vi "Graph.vi"(4 "Resistance":dbl[](array[numeric]), 6 "Array in":T2(array[cluster]), 8 "error in (no error)":errorcluster, 9 "T  (ºC)":dbl format="%.2g", 10 "RH  (%)":dbl format="%.2g", 11 "Ethanol (%)":dbl format="%.3g") -> (0 "error out":errorcluster, 3 "Cluster":T1)   [LabVIEW 2020]
uses:
  typeDefs/Graph.ctl
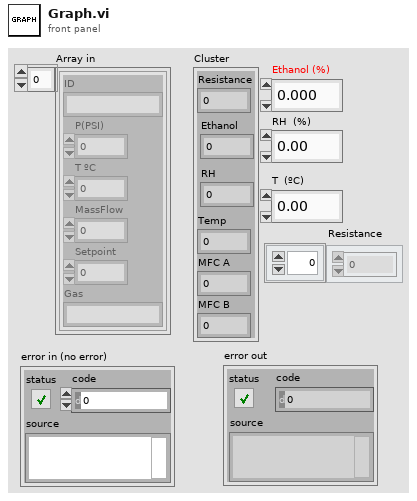
[diagram p1: front panel]
types:
  T1 = typedef "Graph.ctl" = cluster{"Resistance":dbl, "Ethanol":dbl, "RH":dbl, "Temp":dbl, "MFC A":dbl, "MFC B":dbl}
  T2 = cluster{"ID":string, "P(PSI)":dbl, "T ºC":dbl, "MassFlow":dbl, "Setpoint":dbl, "Gas":string}[]
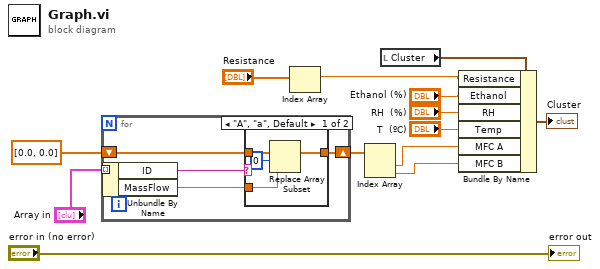
[diagram p0: block diagram]
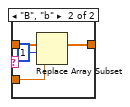
[diagram p2: hidden frame]
diagram:
  n1 = for {
    tunnel: "Array in" -> [w18] mode=indexing
    shift-right: [w15] -> w12
    shift-left: dbl[] [0.0, 0.0] -> [w16]
    n2 = Unbundle By Name(w18) -> ("ID"=w17:string, "MassFlow"=w14:dbl)
    n3 = case shown="\"A\", \"a\", Default" w17 {
      tunnel: [w22 w26] -> w15
      tunnel: w16 -> [w21 w25]
      tunnel: w14 -> [w20 w24]
      frame "A", "a", Default {
        n4 = Replace Array Subset(array=w21, new element=w20, index=0) -> (w22:dbl[])
      }
      frame "B", "b" {
        n5 = Replace Array Subset(array=w25, new element=w24, index=1) -> (w26:dbl[])
      }
    }
  }
  n6 = Index Array(array="Resistance") -> (element=w1:dbl)  [unwired: 1 in]
  n7 = Index Array(array=w12) -> (element #1=w3:dbl, element #2=w13:dbl)  [unwired: 2 in]
  n8 = local read "Cluster"() -> (w4:T1)
  n9 = Bundle By Name(cluster=w4, "Resistance"=w1, "Ethanol"="Ethanol (%)", "RH"="RH  (%)", "Temp"="T  (ºC)", "MFC A"=w3, "MFC B"=w13) -> (→"Cluster":T1)
  "error out" <- "error in (no error)"
